vi "Window Layout.vi"(8 "错误输入":errorcluster caption="错误输入（无错误）") -> (0 "错误输出":errorcluster)   [LabVIEW 2020]
uses:
  <vilib>/Utility/miscctls.llb/LVPointTypeDef.ctl
  <vilib>/Utility/miscctls.llb/LVBoundsTypeDef.ctl
  <vilib>/Utility/miscctls.llb/LVRowAndColumnTypeDef.ctl
panel:
  out "错误输出_处理":errorcluster
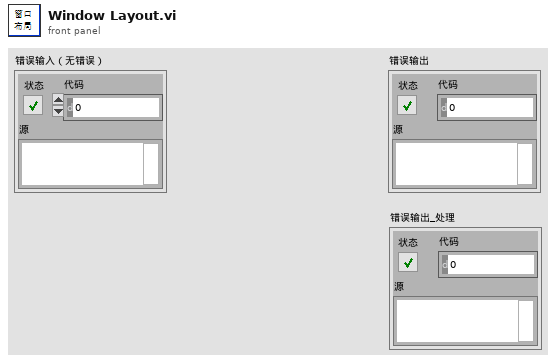
[diagram p1: front panel]
types:
  T1 = typedef "LVPointTypeDef.ctl" = cluster{"Horizontal":i16, "Vertical":i16}
  T2 = enum16{"无", "左边偏移", "右边偏移", "上偏移", "下偏移", "水平居中", "垂直居中", "水平&垂直居中", "匹配窗格"}
  T3 = typedef "LVBoundsTypeDef.ctl" = cluster{"Width":u32, "Height":u32}
  T4 = typedef "LVRowAndColumnTypeDef.ctl" = cluster{"Row":i32, "Column":i32}
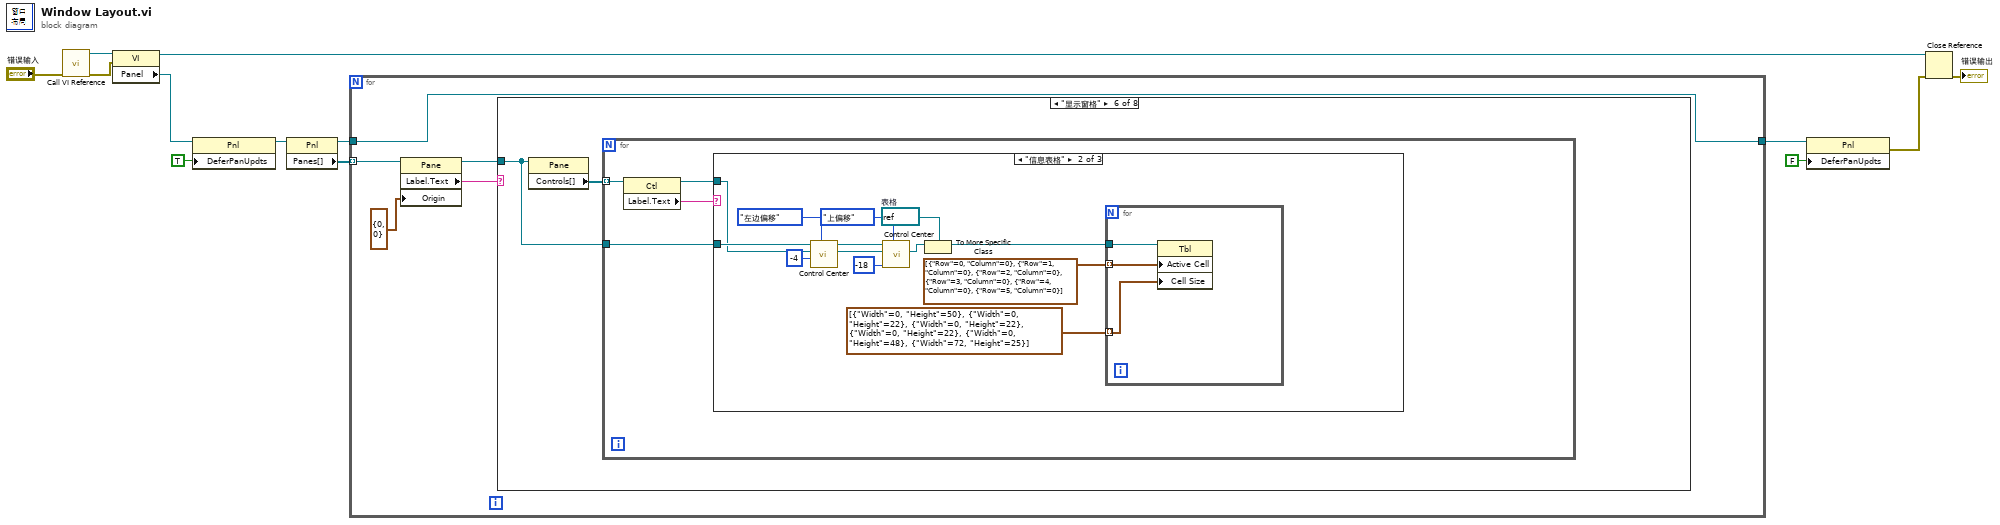
[diagram p0: block diagram]
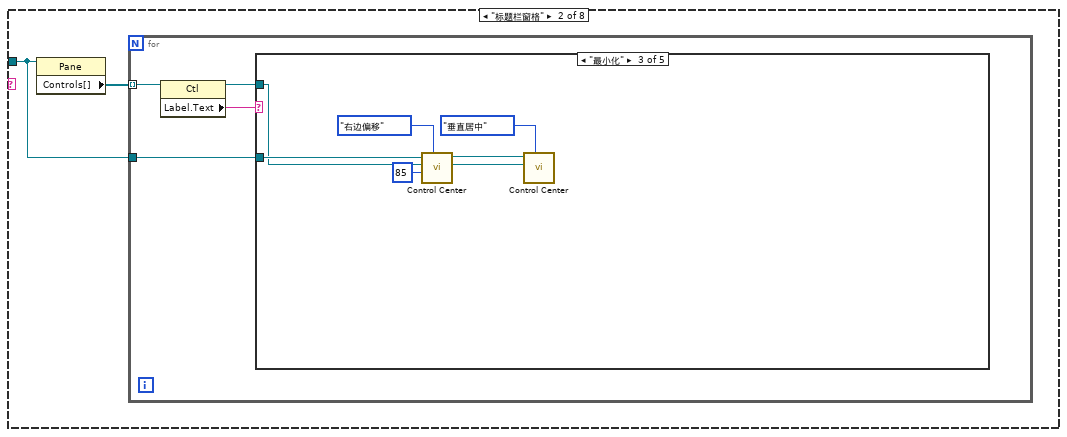
[diagram p3: hidden frame]
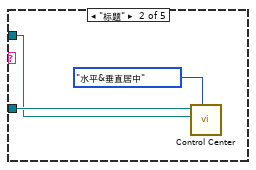
[diagram p5: hidden frame]
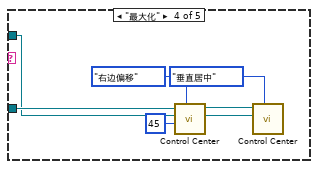
[diagram p6: hidden frame]
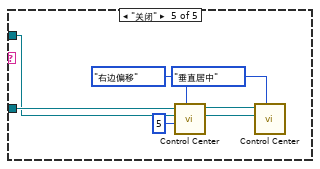
[diagram p7: hidden frame]
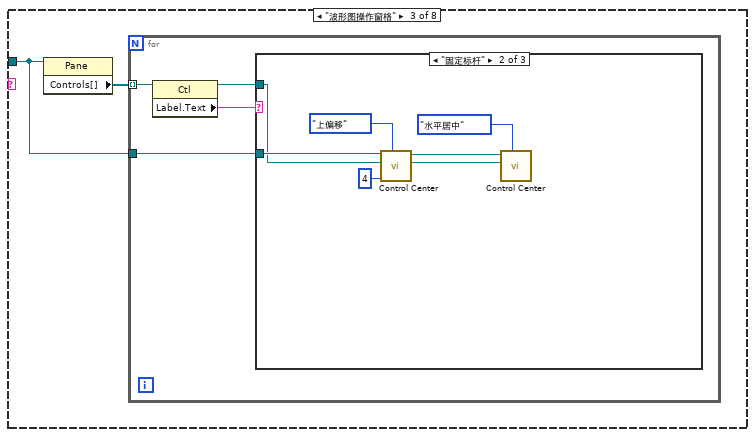
[diagram p8: hidden frame]
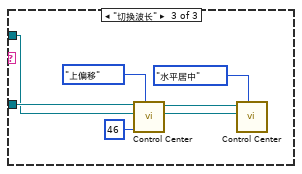
[diagram p10: hidden frame]
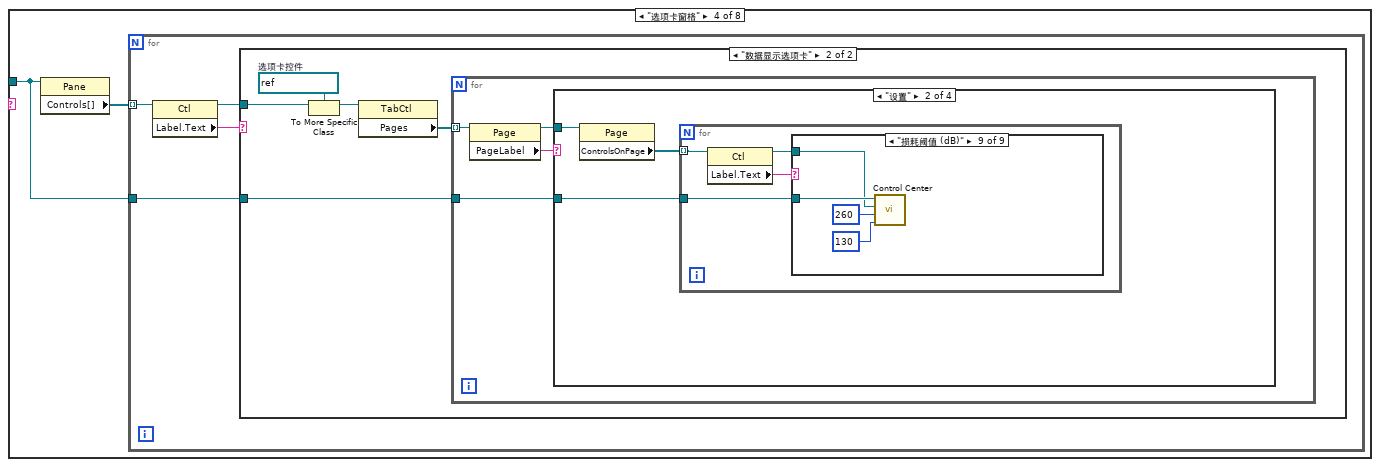
[diagram p11: hidden frame]
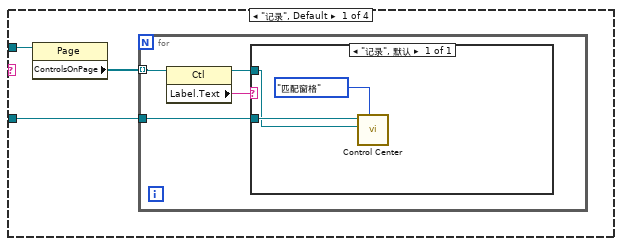
[diagram p13: hidden frame]
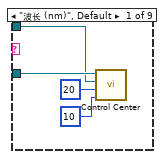
[diagram p14: hidden frame]
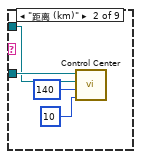
[diagram p15: hidden frame]
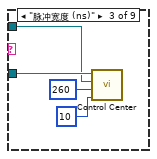
[diagram p16: hidden frame]
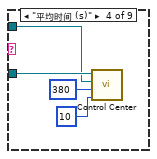
[diagram p17: hidden frame]
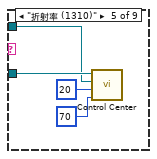
[diagram p18: hidden frame]
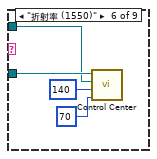
[diagram p19: hidden frame]
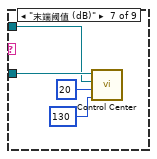
[diagram p20: hidden frame]
diagram:
  n1 = call "Call VI Reference.vi"("error in"="错误输入") -> ("error out"=w2:errorcluster, "vi reference out"=w3:refnum<vi>)  [unwired: 9 in]
  n2 = property class="VI"(reference=w3, error in=w2) -> (reference out=w6:refnum<vi>, "Panel"=w12:refnum<vi>)  [unwired: 1 out]
  n3 = property class="Pnl"(reference=w12, "DeferPanUpdts"=TRUE ("延迟前面板更新")) -> (reference out=w11:refnum<vi>)  [unwired: 1 in, 1 out]
  n4 = property class="Pnl"(reference=w11) -> (reference out=w9:refnum<vi>, "Panes[]"=w13:refnum<vi>[])  [unwired: 1 in, 1 out]
  n5 = for {
    tunnel: w13 -> [w15] mode=indexing
    tunnel: w9 -> [w18]
    tunnel: [w18] -> w8
    n6 = property class="Pane"(reference=w15, "Origin"=T1 {"Horizontal"=0, "Vertical"=0} ("原点")) -> (reference out=w14:refnum<vi>, "Label.Text"=w17:string)  [unwired: 1 in, 1 out]
    n7 = case shown="\"显示窗格\"" w17 {
      tunnel: w14 -> [_ w19 w49 w69 w189 w217 w243 w284]
      frame "eee", Default {
      }
      frame "标题栏窗格" {
        n8 = property class="Pane"(reference=w19) -> ("Controls[]"=w20:refnum<vi>[])  [unwired: 1 in, 2 out]
        n9 = for {
          tunnel: w20 -> [w24] mode=indexing
          tunnel: w19 -> [w21]
          n10 = property class="Ctl"(reference=w24) -> (reference out=w22:refnum<vi>, "Label.Text"=w23:string)  [unwired: 1 in, 1 out]
          n11 = case shown="\"最小化\"" w23 {
            tunnel: w22 -> [_ w26 w33 w40 w47]
            tunnel: w21 -> [_ w27 w34 w41 w48]
            frame "eee", Default {
            }
            frame "标题" {
              n12 = call "Control Center.vi"("Center Style"=T2."水平&垂直居中" ("居中方式"), "Control Re"=w26, "PanelRef"=w27) -> ()  [unwired: 7 in, 2 out]
            }
            frame "最小化" {
              n13 = call "Control Center.vi"("Center Style"=T2."右边偏移" ("居中方式"), "Hor"=85 ("Left"), "Control Re"=w33, "PanelRef"=w34) -> ("Control Ref"=w29:refnum<vi>, "Panel Ref"=w30:refnum<vi>)  [unwired: 6 in]
              n14 = call "Control Center.vi"("Center Style"=T2."垂直居中" ("居中方式"), "Control Re"=w29, "PanelRef"=w30) -> ()  [unwired: 7 in, 2 out]
            }
            frame "最大化" {
              n15 = call "Control Center.vi"("Center Style"=T2."右边偏移" ("居中方式"), "Hor"=45 ("Left"), "Control Re"=w40, "PanelRef"=w41) -> ("Control Ref"=w36:refnum<vi>, "Panel Ref"=w37:refnum<vi>)  [unwired: 6 in]
              n16 = call "Control Center.vi"("Center Style"=T2."垂直居中" ("居中方式"), "Control Re"=w36, "PanelRef"=w37) -> ()  [unwired: 7 in, 2 out]
            }
            frame "关闭" {
              n17 = call "Control Center.vi"("Center Style"=T2."右边偏移" ("居中方式"), "Hor"=5 ("Left"), "Control Re"=w47, "PanelRef"=w48) -> ("Control Ref"=w43:refnum<vi>, "Panel Ref"=w44:refnum<vi>)  [unwired: 6 in]
              n18 = call "Control Center.vi"("Center Style"=T2."垂直居中" ("居中方式"), "Control Re"=w43, "PanelRef"=w44) -> ()  [unwired: 7 in, 2 out]
            }
          }
        }
      }
      frame "波形图操作窗格" {
        n19 = property class="Pane"(reference=w49) -> ("Controls[]"=w50:refnum<vi>[])  [unwired: 1 in, 2 out]
        n20 = for {
          tunnel: w50 -> [w54] mode=indexing
          tunnel: w49 -> [w51]
          n21 = property class="Ctl"(reference=w54) -> (reference out=w52:refnum<vi>, "Label.Text"=w53:string)  [unwired: 1 in, 1 out]
          n22 = case shown="\"固定标杆\"" w53 {
            tunnel: w52 -> [_ w60 w67]
            tunnel: w51 -> [_ w61 w68]
            frame "eee", Default {
            }
            frame "固定标杆" {
              n23 = call "Control Center.vi"("Center Style"=T2."上偏移" ("居中方式"), "Vertical"=4 ("Top"), "Control Re"=w60, "PanelRef"=w61) -> ("Control Ref"=w55:refnum<vi>, "Panel Ref"=w56:refnum<vi>)  [unwired: 6 in]
              n24 = call "Control Center.vi"("Center Style"=T2."水平居中" ("居中方式"), "Control Re"=w55, "PanelRef"=w56) -> ()  [unwired: 7 in, 2 out]
            }
            frame "切换波长" {
              n25 = call "Control Center.vi"("Center Style"=T2."上偏移" ("居中方式"), "Vertical"=46 ("Top"), "Control Re"=w67, "PanelRef"=w68) -> ("Control Ref"=w62:refnum<vi>, "Panel Ref"=w63:refnum<vi>)  [unwired: 6 in]
              n26 = call "Control Center.vi"("Center Style"=T2."水平居中" ("居中方式"), "Control Re"=w62, "PanelRef"=w63) -> ()  [unwired: 7 in, 2 out]
            }
          }
        }
      }
      frame "选项卡窗格" {
        n27 = property class="Pane"(reference=w69) -> ("Controls[]"=w70:refnum<vi>[])  [unwired: 1 in, 2 out]
        n28 = for {
          tunnel: w70 -> [w74] mode=indexing
          tunnel: w69 -> [w71]
          n29 = property class="Ctl"(reference=w74) -> (reference out=w73:refnum<vi>, "Label.Text"=w72:string)  [unwired: 1 in, 1 out]
          n30 = case shown="\"数据显示选项卡\"" w72 {
            tunnel: w73 -> [_ w78]
            tunnel: w71 -> [_ w75]
            frame "eee", Default {
            }
            frame "数据显示选项卡" {
              w77 = refnum<vi> refnum  # 选项卡控件
              n31 = To More Specific Class(target class=w77, reference=w78) -> (specific class reference=w76:refnum<vi>)  [unwired: 1 in, 1 out]
              n32 = property class="TabCtl"(reference=w76) -> ("Pages"=w79:refnum<vi>[])  [unwired: 1 in, 2 out]
              n33 = for {
                tunnel: w79 -> [w83] mode=indexing
                tunnel: w75 -> [w80]
                n34 = property class="Page"(reference=w83) -> (reference out=w81:refnum<vi>, "PageLabel"=w82:string)  [unwired: 1 in, 1 out]
                n35 = case shown="\"设置\"" w82 {
                  tunnel: w81 -> [w85 w95 w139 w149]
                  tunnel: w80 -> [w84 w94 w137 w147]
                  frame "记录", Default {
                    n36 = property class="Page"(reference=w85) -> ("ControlsOnPage"=w86:refnum<vi>[])  [unwired: 1 in, 2 out]
                    n37 = for {
                      tunnel: w86 -> [w90] mode=indexing
                      tunnel: w84 -> [w87]
                      n38 = property class="Ctl"(reference=w90) -> (reference out=w88:refnum<vi>, "Label.Text"=w89:string)  [unwired: 1 in, 1 out]
                      n39 = case shown="\"记录\", 默认" w89 {
                        tunnel: w88 -> [w92]
                        tunnel: w87 -> [w93]
                        frame "记录", Default {
                          n40 = call "Control Center.vi"("Center Style"=T2."匹配窗格" ("居中方式"), "Control Re"=w92, "PanelRef"=w93) -> ()  [unwired: 7 in, 2 out]
                        }
                      }
                    }
                  }
                  frame "设置" {
                    n41 = property class="Page"(reference=w95) -> ("ControlsOnPage"=w96:refnum<vi>[])  [unwired: 1 in, 2 out]
                    n42 = for {
                      tunnel: w96 -> [w100] mode=indexing
                      tunnel: w94 -> [w97]
                      n43 = property class="Ctl"(reference=w100) -> (reference out=w98:refnum<vi>, "Label.Text"=w99:string)  [unwired: 1 in, 1 out]
                      n44 = case shown="\"损耗阈值 (dB)\"" w99 {
                        tunnel: w98 -> [w103 w107 w111 w115 w119 w123 w127 w131 w135]
                        tunnel: w97 -> [w104 w108 w112 w116 w120 w124 w128 w132 w136]
                        frame "波长 (nm)", Default {
                          n45 = call "Control Center.vi"("Vertical"=10 ("Top"), "Hor"=20 ("Left"), "Control Re"=w103, "PanelRef"=w104) -> ()  [unwired: 6 in, 2 out]
                        }
                        frame "距离 (km)" {
                          n46 = call "Control Center.vi"("Vertical"=10 ("Top"), "Hor"=140 ("Left"), "Control Re"=w107, "PanelRef"=w108) -> ()  [unwired: 6 in, 2 out]
                        }
                        frame "脉冲宽度 (ns)" {
                          n47 = call "Control Center.vi"("Vertical"=10 ("Top"), "Hor"=260 ("Left"), "Control Re"=w111, "PanelRef"=w112) -> ()  [unwired: 6 in, 2 out]
                        }
                        frame "平均时间 (s)" {
                          n48 = call "Control Center.vi"("Vertical"=10 ("Top"), "Hor"=380 ("Left"), "Control Re"=w115, "PanelRef"=w116) -> ()  [unwired: 6 in, 2 out]
                        }
                        frame "折射率 (1310)" {
                          n49 = call "Control Center.vi"("Vertical"=70 ("Top"), "Hor"=20 ("Left"), "Control Re"=w119, "PanelRef"=w120) -> ()  [unwired: 6 in, 2 out]
                        }
                        frame "折射率 (1550)" {
                          n50 = call "Control Center.vi"("Vertical"=70 ("Top"), "Hor"=140 ("Left"), "Control Re"=w123, "PanelRef"=w124) -> ()  [unwired: 6 in, 2 out]
                        }
                        frame "末端阈值 (dB)" {
                          n51 = call "Control Center.vi"("Vertical"=130 ("Top"), "Hor"=20 ("Left"), "Control Re"=w127, "PanelRef"=w128) -> ()  [unwired: 6 in, 2 out]
                        }
                        frame "反射阈值 (dB)" {
                          n52 = call "Control Center.vi"("Vertical"=130 ("Top"), "Hor"=140 ("Left"), "Control Re"=w131, "PanelRef"=w132) -> ()  [unwired: 6 in, 2 out]
                        }
                        frame "损耗阈值 (dB)" {
                          n53 = call "Control Center.vi"("Vertical"=130 ("Top"), "Hor"=260 ("Left"), "Control Re"=w135, "PanelRef"=w136) -> ()  [unwired: 6 in, 2 out]
                        }
                      }
                    }
                  }
                  frame "事件" {
                    n54 = property class="Page"(reference=w139) -> ("ControlsOnPage"=w138:refnum<vi>[])  [unwired: 1 in, 2 out]
                    n55 = for {
                      tunnel: w138 -> [w143] mode=indexing
                      tunnel: w137 -> [w140]
                      n56 = property class="Ctl"(reference=w143) -> (reference out=w141:refnum<vi>, "Label.Text"=w142:string)  [unwired: 1 in, 1 out]
                      n57 = case shown="\"事件信息\", 默认" w142 {
                        tunnel: w141 -> [w146]
                        tunnel: w140 -> [w145]
                        frame "事件信息", Default {
                          n58 = call "Control Center.vi"("Center Style"=T2."匹配窗格" ("居中方式"), "Control Re"=w146, "PanelRef"=w145) -> ()  [unwired: 7 in, 2 out]
                        }
                      }
                    }
                  }
                  frame "分析" {
                    n59 = property class="Page"(reference=w149) -> ("ControlsOnPage"=w148:refnum<vi>[])  [unwired: 1 in, 2 out]
                    n60 = for {
                      tunnel: w148 -> [w156] mode=indexing
                      tunnel: w147 -> [w152]
                      n61 = property class="Pane"(reference=w152) -> (reference out=w151:refnum<vi>, "Bounds"=w150:T3)  [unwired: 1 in, 1 out]
                      n62 = property class="Ctl"(reference=w156) -> (reference out=w154:refnum<vi>, "Label.Text"=w155:string)  [unwired: 1 in, 1 out]
                      n63 = case shown="\"文件列表\", 默认" w155 {
                        tunnel: w154 -> [w170 w187]
                        tunnel: [w166 w184] -> w153
                        tunnel: w151 -> [w162 w173]
                        tunnel: w150 -> [w165 w181]
                        frame "文件列表", Default {
                          w171 = refnum<vi> refnum  # 多列列表框
                          n64 = To More Specific Class(target class=w171, reference=w170) -> (specific class reference=w169:refnum<vi>, error out=w168:errorcluster)  [unwired: 1 in]
                          n65 = Subtract(x=w165, y=T3 {"Width"=4, "Height"=32}) -> (x-y=w164:T3)
                          n66 = property class="MCListbox"(reference=w169, error in=w168, "Size"=w164) -> (reference out=w163:refnum<vi>, error out=w166:errorcluster)
                          n67 = call "Control Center.vi"("Center Style"=T2."水平居中" ("居中方式"), "Control Re"=w163, "PanelRef"=w162) -> ("Control Ref"=w159:refnum<vi>, "Panel Ref"=w160:refnum<vi>)  [unwired: 7 in]
                          n68 = call "Control Center.vi"("Center Style"=T2."上偏移" ("居中方式"), "Vertical"=2 ("垂直"), "Control Re"=w159, "PanelRef"=w160) -> ()  [unwired: 6 in, 2 out]
                        }
                        frame "文件夹路径" {
                          w188 = refnum<vi> refnum  # 路径
                          n69 = Unbundle By Name(w181) -> ("Width"=w183:u32)
                          n70 = To More Specific Class(target class=w188, reference=w187) -> (specific class reference=w186:refnum<vi>, error out=w185:errorcluster)  [unwired: 1 in]
                          n71 = Subtract(x=w183, y=u32 30 ("Height")) -> (x-y=w180:u32)
                          n72 = property class="Path"(reference=w186, error in=w185, "Height"=u32 25 ("大小:高度"), "Width"=w180) -> (reference out=w172:refnum<vi>, error out=w184:errorcluster)
                          n73 = call "Control Center.vi"("Center Style"=T2."水平居中" ("居中方式"), "Control Re"=w172, "PanelRef"=w173) -> ("Control Ref"=w175:refnum<vi>, "Panel Ref"=w176:refnum<vi>)  [unwired: 7 in]
                          n74 = call "Control Center.vi"("Center Style"=T2."下偏移" ("居中方式"), "Vertical"=2 ("垂直"), "Control Re"=w175, "PanelRef"=w176) -> ()  [unwired: 6 in, 2 out]
                        }
                      }
                      "错误输出_处理" <- w153
                    }
                  }
                }
              }
            }
          }
        }
      }
      frame "选项卡操作窗格" {
        n75 = property class="Pane"(reference=w189) -> ("Controls[]"=w190:refnum<vi>[])  [unwired: 1 in, 2 out]
        n76 = for {
          tunnel: w190 -> [w195] mode=indexing
          tunnel: w189 -> [w191]
          n77 = property class="Ctl"(reference=w195) -> (reference out=w193:refnum<vi>, "Label.Text"=w194:string, "Bounds"=w192:T3)  [unwired: 1 in, 1 out]
          n78 = case shown="\"设置\"" w194 {
            tunnel: w193 -> [_ w201 w208 w215]
            tunnel: w192 -> [_ _ _ _]
            tunnel: w191 -> [_ w202 w209 w216]
            frame "eee", Default {
            }
            frame "设置" {
              n79 = call "Control Center.vi"("Center Style"=T2."左边偏移" ("居中方式"), "Hor"=3 ("Left"), "Control Re"=w201, "PanelRef"=w202) -> ("Control Ref"=w198:refnum<vi>, "Panel Ref"=w199:refnum<vi>)  [unwired: 6 in]
              n80 = call "Control Center.vi"("Center Style"=T2."垂直居中" ("居中方式"), "Control Re"=w198, "PanelRef"=w199) -> ()  [unwired: 7 in, 2 out]
            }
            frame "事件" {
              n81 = call "Control Center.vi"("Center Style"=T2."左边偏移" ("居中方式"), "Hor"=86 ("Left"), "Control Re"=w208, "PanelRef"=w209) -> ("Control Ref"=w204:refnum<vi>, "Panel Ref"=w205:refnum<vi>)  [unwired: 6 in]
              n82 = call "Control Center.vi"("Center Style"=T2."垂直居中" ("居中方式"), "Control Re"=w204, "PanelRef"=w205) -> ()  [unwired: 7 in, 2 out]
            }
            frame "分析" {
              n83 = call "Control Center.vi"("Center Style"=T2."左边偏移" ("居中方式"), "Hor"=169 ("Left"), "Control Re"=w215, "PanelRef"=w216) -> ("Control Ref"=w211:refnum<vi>, "Panel Ref"=w212:refnum<vi>)  [unwired: 6 in]
              n84 = call "Control Center.vi"("Center Style"=T2."垂直居中" ("居中方式"), "Control Re"=w211, "PanelRef"=w212) -> ()  [unwired: 7 in, 2 out]
            }
          }
        }
      }
      frame "显示窗格" {
        n85 = property class="Pane"(reference=w217) -> ("Controls[]"=w218:refnum<vi>[])  [unwired: 1 in, 2 out]
        n86 = for {
          tunnel: w218 -> [w222] mode=indexing
          tunnel: w217 -> [w219]
          n87 = property class="Ctl"(reference=w222) -> (reference out=w220:refnum<vi>, "Label.Text"=w221:string)  [unwired: 1 in, 1 out]
          n88 = case shown="\"信息表格\"" w221 {
            tunnel: w220 -> [_ w234 w241]
            tunnel: w219 -> [_ w235 w242]
            frame "eee", Default {
            }
            frame "信息表格" {
              w227 = refnum<vi> refnum  # 表格
              n89 = call "Control Center.vi"("Center Style"=T2."左边偏移" ("居中方式"), "Hor"=-4 ("水平"), "Control Re"=w234, "PanelRef"=w235) -> ("Control Ref"=w231:refnum<vi>, "Panel Ref"=w232:refnum<vi>)  [unwired: 6 in]
              n90 = call "Control Center.vi"("Center Style"=T2."上偏移" ("居中方式"), "Vertical"=-18 ("垂直"), "Control Re"=w231, "PanelRef"=w232) -> ("Control Ref"=w223:refnum<vi>)  [unwired: 6 in, 1 out]
              n91 = To More Specific Class(target class=w227, reference=w223) -> (specific class reference=w226:refnum<vi>)  [unwired: 1 in, 1 out]
              n92 = for {
                tunnel: w226 -> [w238]
                tunnel: T4[] [{"Row"=0, "Column"=0}, {"Row"=1, "Column"=0}, {"Row"=2, "Column"=0}, {"Row"=3, "Column"=0}, {"Row"=4, "Column"=0}, {"Row"=5, "Column"=0}] ("活动单元格:活动单元格") -> [w237] mode=indexing
                tunnel: T3[] [{"Width"=0, "Height"=50}, {"Width"=0, "Height"=22}, {"Width"=0, "Height"=22}, {"Width"=0, "Height"=22}, {"Width"=0, "Height"=48}, {"Width"=72, "Height"=25}] ("活动单元格:单元格大小") -> [w236] mode=indexing
                n93 = property class="Tbl"(reference=w238, "Active Cell"=w237, "Cell Size"=w236) -> ()  [unwired: 1 in, 2 out]
              }
            }
            frame "当前波长" {
              n94 = call "Control Center.vi"("Center Style"=T2."水平居中" ("居中方式"), "Vertical"=0 ("垂直"), "Control Re"=w241, "PanelRef"=w242) -> ()  [unwired: 6 in, 2 out]
            }
          }
        }
      }
      frame "菜单栏窗格" {
        n95 = property class="Pane"(reference=w243) -> ("Controls[]"=w244:refnum<vi>[])  [unwired: 1 in, 2 out]
        n96 = for {
          tunnel: w244 -> [w248] mode=indexing
          tunnel: w243 -> [w245]
          n97 = property class="Ctl"(reference=w248) -> (reference out=w246:refnum<vi>, "Label.Text"=w247:string)  [unwired: 1 in, 1 out]
          n98 = case shown="\"保存数据\"" w247 {
            tunnel: w246 -> [_ w254 w261 w268 w275 w282]
            tunnel: w245 -> [_ w255 w262 w269 w276 w283]
            frame "eee", Default {
            }
            frame "手动连接" {
              n99 = call "Control Center.vi"("Center Style"=T2."上偏移" ("居中方式"), "Vertical"=6 ("Top"), "Control Re"=w254, "PanelRef"=w255) -> ("Control Ref"=w249:refnum<vi>, "Panel Ref"=w250:refnum<vi>)  [unwired: 6 in]
              n100 = call "Control Center.vi"("Center Style"=T2."水平居中" ("居中方式"), "Control Re"=w249, "PanelRef"=w250) -> ()  [unwired: 7 in, 2 out]
            }
            frame "实时测量" {
              n101 = call "Control Center.vi"("Center Style"=T2."上偏移" ("居中方式"), "Vertical"=66 ("Top"), "Control Re"=w261, "PanelRef"=w262) -> ("Control Ref"=w256:refnum<vi>, "Panel Ref"=w257:refnum<vi>)  [unwired: 6 in]
              n102 = call "Control Center.vi"("Center Style"=T2."水平居中" ("居中方式"), "Control Re"=w256, "PanelRef"=w257) -> ()  [unwired: 7 in, 2 out]
            }
            frame "自动测量" {
              n103 = call "Control Center.vi"("Center Style"=T2."上偏移" ("居中方式"), "Vertical"=126 ("Top"), "Control Re"=w268, "PanelRef"=w269) -> ("Control Ref"=w264:refnum<vi>, "Panel Ref"=w265:refnum<vi>)  [unwired: 6 in]
              n104 = call "Control Center.vi"("Center Style"=T2."水平居中" ("居中方式"), "Control Re"=w264, "PanelRef"=w265) -> ()  [unwired: 7 in, 2 out]
            }
            frame "停止测量" {
              n105 = call "Control Center.vi"("Center Style"=T2."上偏移" ("居中方式"), "Vertical"=186 ("Top"), "Control Re"=w275, "PanelRef"=w276) -> ("Control Ref"=w271:refnum<vi>, "Panel Ref"=w272:refnum<vi>)  [unwired: 6 in]
              n106 = call "Control Center.vi"("Center Style"=T2."水平居中" ("居中方式"), "Control Re"=w271, "PanelRef"=w272) -> ()  [unwired: 7 in, 2 out]
            }
            frame "保存数据" {
              n107 = call "Control Center.vi"("Center Style"=T2."上偏移" ("居中方式"), "Vertical"=246 ("Top"), "Control Re"=w282, "PanelRef"=w283) -> ("Control Ref"=w278:refnum<vi>, "Panel Ref"=w279:refnum<vi>)  [unwired: 6 in]
              n108 = call "Control Center.vi"("Center Style"=T2."水平居中" ("居中方式"), "Control Re"=w278, "PanelRef"=w279) -> ()  [unwired: 7 in, 2 out]
            }
          }
        }
      }
      frame "任务栏窗格" {
        n109 = property class="Pane"(reference=w284) -> ("Controls[]"=w285:refnum<vi>[])  [unwired: 1 in, 2 out]
        n110 = for {
          tunnel: w285 -> [w289] mode=indexing
          tunnel: w284 -> [w286]
          n111 = property class="Ctl"(reference=w289) -> (reference out=w287:refnum<vi>, "Label.Text"=w288:string)  [unwired: 1 in, 1 out]
          n112 = case shown="\"连接\"" w288 {
            tunnel: w287 -> [_ w295 w302 w309 w316 w323]
            tunnel: w286 -> [_ w296 w303 w310 w317 w324]
            frame "eee", Default {
            }
            frame "参数显示" {
              n113 = call "Control Center.vi"("Center Style"=T2."左边偏移" ("居中方式"), "Hor"=2 ("Left"), "Control Re"=w295, "PanelRef"=w296) -> ("Control Ref"=w291:refnum<vi>, "Panel Ref"=w292:refnum<vi>)  [unwired: 6 in]
              n114 = call "Control Center.vi"("Center Style"=T2."垂直居中" ("居中方式"), "Control Re"=w291, "PanelRef"=w292) -> ()  [unwired: 7 in, 2 out]
            }
            frame "保存" {
              n115 = call "Control Center.vi"("Center Style"=T2."右边偏移" ("居中方式"), "Hor"=310 ("Left"), "Control Re"=w302, "PanelRef"=w303) -> ("Control Ref"=w298:refnum<vi>, "Panel Ref"=w299:refnum<vi>)  [unwired: 6 in]
              n116 = call "Control Center.vi"("Center Style"=T2."垂直居中" ("居中方式"), "Control Re"=w298, "PanelRef"=w299) -> ()  [unwired: 7 in, 2 out]
            }
            frame "连接" {
              n117 = call "Control Center.vi"("Center Style"=T2."右边偏移" ("居中方式"), "Hor"=250 ("Left"), "Control Re"=w309, "PanelRef"=w310) -> ("Control Ref"=w305:refnum<vi>, "Panel Ref"=w306:refnum<vi>)  [unwired: 6 in]
              n118 = call "Control Center.vi"("Center Style"=T2."垂直居中" ("居中方式"), "Control Re"=w305, "PanelRef"=w306) -> ()  [unwired: 7 in, 2 out]
            }
            frame "进度条" {
              n119 = call "Control Center.vi"("Center Style"=T2."右边偏移" ("居中方式"), "Hor"=136 ("Left"), "Control Re"=w316, "PanelRef"=w317) -> ("Control Ref"=w312:refnum<vi>, "Panel Ref"=w313:refnum<vi>)  [unwired: 6 in]
              n120 = call "Control Center.vi"("Center Style"=T2."垂直居中" ("居中方式"), "Control Re"=w312, "PanelRef"=w313) -> ()  [unwired: 7 in, 2 out]
            }
            frame "时间日期" {
              n121 = call "Control Center.vi"("Center Style"=T2."右边偏移" ("居中方式"), "Hor"=3 ("Left"), "Control Re"=w323, "PanelRef"=w324) -> ("Control Ref"=w319:refnum<vi>, "Panel Ref"=w320:refnum<vi>)  [unwired: 6 in]
              n122 = call "Control Center.vi"("Center Style"=T2."垂直居中" ("居中方式"), "Control Re"=w319, "PanelRef"=w320) -> ()  [unwired: 7 in, 2 out]
            }
          }
        }
      }
    }
  }
  n123 = property class="Pnl"(reference=w8, "DeferPanUpdts"=FALSE ("延迟前面板更新")) -> (error out=w5:errorcluster)  [unwired: 1 in, 1 out]
  n124 = Close Reference(reference=w6, error in (no error)=w5) -> (error out=→"错误输出":errorcluster)
